vi "MSEditor_Script_GetHeaderParam.vi"(0 "Script refnum":refnum<vi>) -> (1 "Name":string, 2 "Version":string)   [LabVIEW 2018]
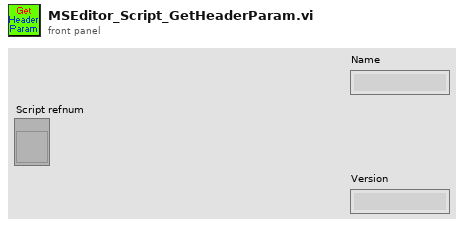
[diagram p1: front panel]
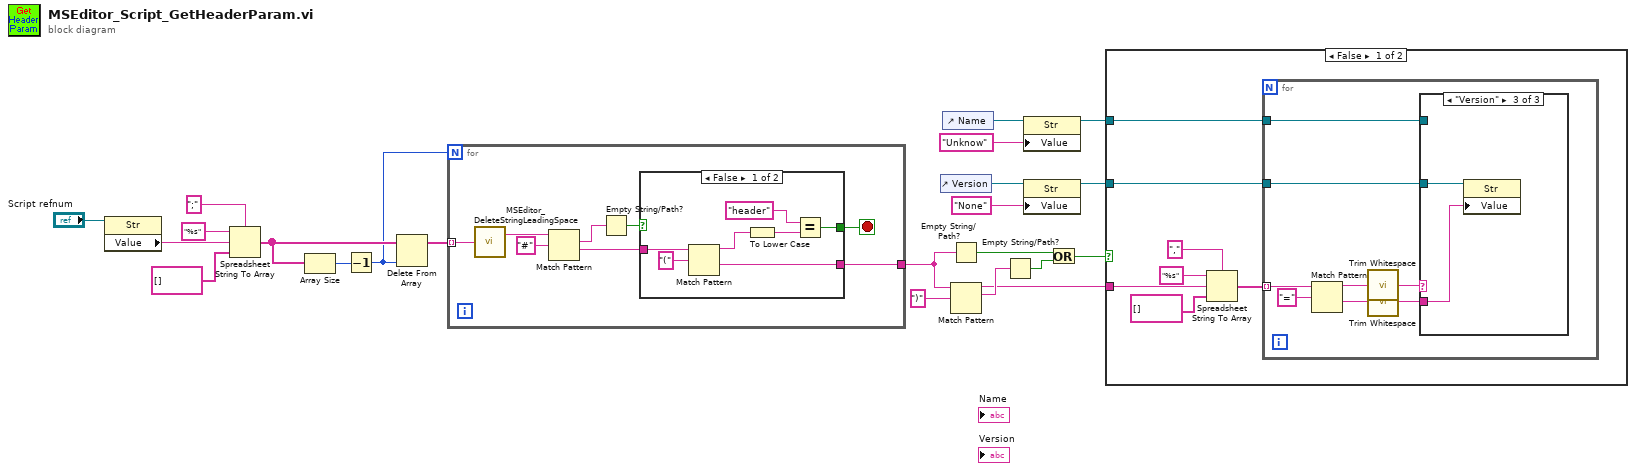
[diagram p0: block diagram]
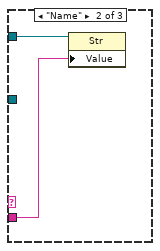
[diagram p3: hidden frame]
diagram:
  n1 = property class="Str"(reference="Script refnum") -> ("Value"=w7:string)  [unwired: 1 in, 2 out]
  n2 = Spreadsheet String To Array(delimiter (Tab)=";", format string="%s", spreadsheet string=w7, array type (2D Dbl)=string[] []) -> (array=w19:string[])
  n3 = Array Size(array=w19) -> (size(s)=w18:i32)
  n4 = Decrement(x=w18) -> (x-1=w16:i32)
  n5 = Delete From Array(array=w19, index=w16) -> (array with subset deleted=w17:string[])  [unwired: 1 in, 1 out]
  n6 = for {
    N: w16 -> [_]
    tunnel: w17 -> [w30] mode=indexing
    tunnel: [w23] -> w14
    stop <- w24 stop-if-true
    n7 = call "MSEditor_DeleteStringLeadingSpace.vi"("string in"=w30) -> ("string after leading space"=w27:string)  [unwired: 1 out]
    n8 = Match Pattern(string=w27, regular expression="#") -> (match substring=w29:string, after substring=w25:string)  [unwired: 1 in, 2 out]
    n9 = Empty String/Path?(string/path=w29) -> (empty?=w26:bool)
    n10 = case shown="False" w26 {
      tunnel: w25 -> [w36 _]
      tunnel: [w32 _] -> w24
      tunnel: [w31 _] -> w23
      frame False {
        n11 = Match Pattern(string=w36, regular expression="(") -> (before substring=w35:string, after substring=w31:string)  [unwired: 1 in, 2 out]
        n12 = To Lower Case(string=w35) -> (all lower case string=w33:string)
        n13 = Equal?(x="header" ("string"), y=w33) -> (x = y?=w32:bool)
      }
      frame True {
      }
    }
  }
  n14 = control-ref of="Version"() -> (w5:refnum<vi>)
  n15 = control-ref of="Name"() -> (w6:refnum<vi>)
  n16 = Empty String/Path?(string/path=w14) -> (empty?=w13:bool)
  n17 = Match Pattern(string=w14, regular expression=")") -> (before substring=w9:string, match substring=w10:string)  [unwired: 1 in, 2 out]
  n18 = Empty String/Path?(string/path=w10) -> (empty?=w12:bool)
  n19 = property class="Str"(reference=w6, "Value"="Unknow") -> (reference out=w1:refnum<vi>)  [unwired: 1 in, 1 out]
  n20 = property class="Str"(reference=w5, "Value"="None") -> (reference out=w2:refnum<vi>)  [unwired: 1 in, 1 out]
  n21 = Or(x=w13, y=w12) -> (x .or. y?=w11:bool)
  n22 = case shown="False" w11 {
    tunnel: w9 -> [w42 _]
    tunnel: w2 -> [w39 _]
    tunnel: w1 -> [w38 _]
    frame False {
      n23 = Spreadsheet String To Array(delimiter (Tab)=",", format string="%s", spreadsheet string=w42, array type (2D Dbl)=string[] []) -> (array=w40:string[])
      n24 = for {
        tunnel: w40 -> [w51] mode=indexing
        tunnel: w39 -> [w50]
        tunnel: w38 -> [w49]
        n25 = Match Pattern(string=w51, regular expression="=") -> (before substring=w48:string, after substring=w46:string)  [unwired: 1 in, 2 out]
        n26 = call <vilib>:"Trim Whitespace.vi"("string"=w48) -> ("trimmed string"=w47:string)  [unwired: 1 in]
        n27 = call <vilib>:"Trim Whitespace.vi"("string"=w46) -> ("trimmed string"=w45:string)  [unwired: 1 in]
        n28 = case shown="\"Version\"" w47 {
          tunnel: w49 -> [_ w54 _]
          tunnel: w50 -> [_ _ w55]
          tunnel: w45 -> [_ w53 w56]
          frame "False", Default {
          }
          frame "Name" {
            n29 = property class="Str"(reference=w54, "Value"=w53) -> ()  [unwired: 1 in, 2 out]
          }
          frame "Version" {
            n30 = property class="Str"(reference=w55, "Value"=w56) -> ()  [unwired: 1 in, 2 out]
          }
        }
      }
    }
    frame True {
    }
  }
